vi "String To Float_csm.vi"(2 "Default (0)":dbl, 5 "String":string) -> (0 "Float":dbl format="%.2p", 1 "Unit String":string)   [LabVIEW 2017, in "API String Arguments Support.lvlib"]
uses:
  API String Arguments Support.lvlib
  <userlib>/_NEVSTOP/Communicable State Machine(CSM)/_Shared/CSM Shared.lvlib
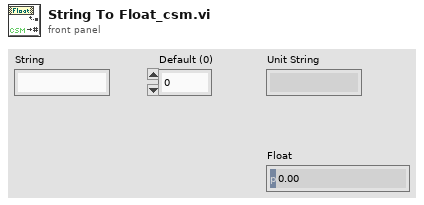
[diagram p1: front panel]
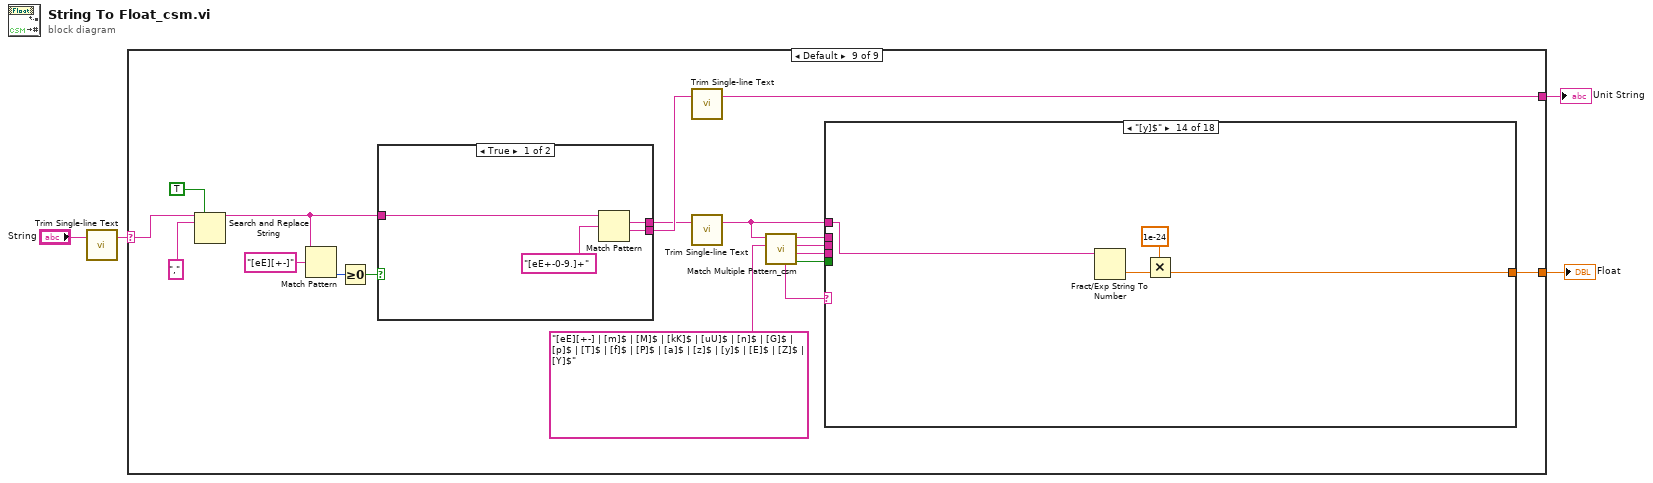
[diagram p0: block diagram]
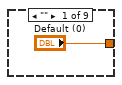
[diagram p2: hidden frame]
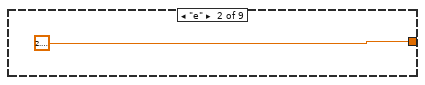
[diagram p3: hidden frame]
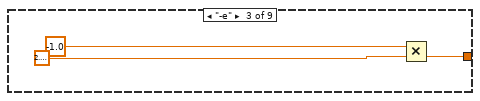
[diagram p4: hidden frame]
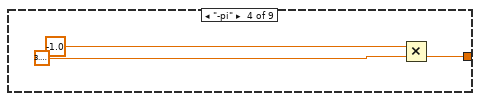
[diagram p5: hidden frame]
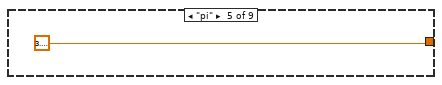
[diagram p6: hidden frame]
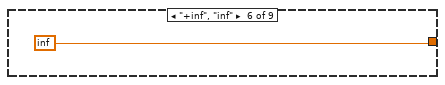
[diagram p7: hidden frame]
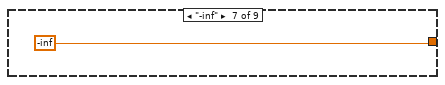
[diagram p8: hidden frame]
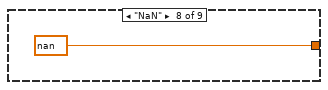
[diagram p9: hidden frame]
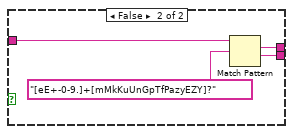
[diagram p10: hidden frame]
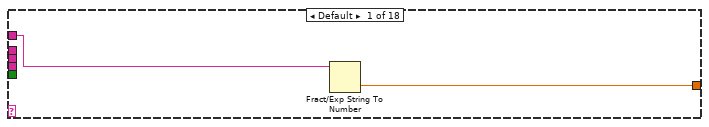
[diagram p11: hidden frame]
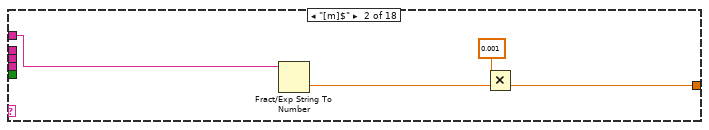
[diagram p12: hidden frame]
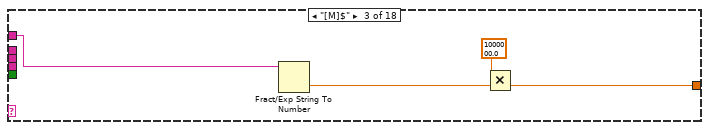
[diagram p13: hidden frame]
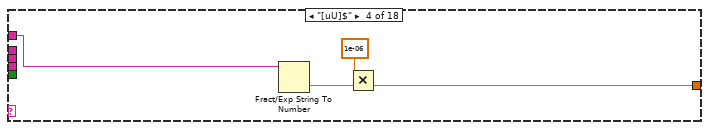
[diagram p14: hidden frame]
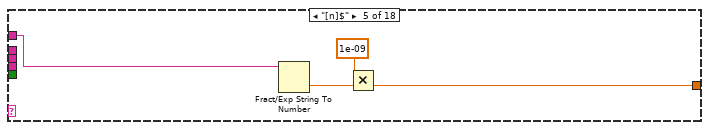
[diagram p15: hidden frame]
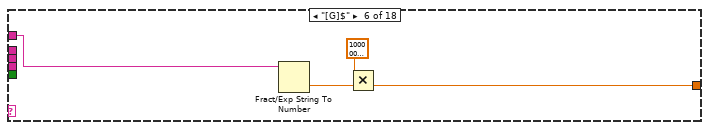
[diagram p16: hidden frame]
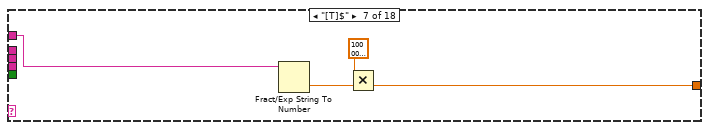
[diagram p17: hidden frame]
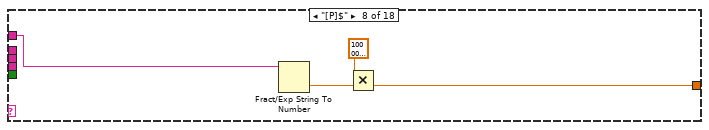
[diagram p18: hidden frame]
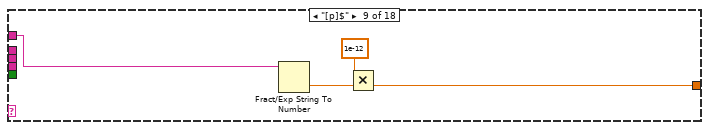
[diagram p19: hidden frame]
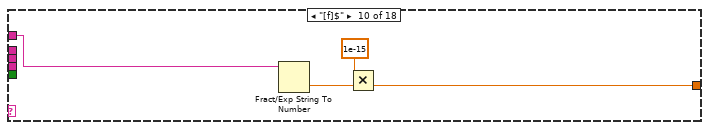
[diagram p20: hidden frame]
diagram:
  n1 = call <userlib>:"Trim Single-line Text.vi"("single-line text"="String") -> ("trimed text"=w2:string)  [unwired: 2 in]
  n2 = case shown="Default" w2 {
    selector: w2 -> [_ _ _ _ _ _ _ _ w25]
    tunnel: ["Default (0)" 2.718281828459045 w8 w11 3.141592653589793 inf -inf nan ("Default(0)") w27] -> w3
    tunnel: [_ _ _ _ _ _ _ _ w23] -> w1
    frame "" {
    }
    frame "e" {
    }
    frame "-e" {
      n3 = Multiply(x=-1.0, y=2.718281828459045) -> (x*y=w8:dbl)
    }
    frame "-pi" {
      n4 = Multiply(x=-1.0, y=3.141592653589793) -> (x*y=w11:dbl)
    }
    frame "pi" {
    }
    frame "+inf", "inf" {
    }
    frame "-inf" {
    }
    frame "NaN" {
    }
    frame Default {
      n5 = Search and Replace String(replace all?=TRUE ("replace all? (F)"), input string=w25, search string=",") -> (result string=w19:string)  [unwired: 5 in, 3 out]
      n6 = Match Pattern(string=w19, regular expression="[eE][+-]") -> (offset past match=w18:i32)  [unwired: 1 in, 3 out]
      n7 = Greater Or Equal To 0?(x=w18) -> (x >= 0?=w17:bool)
      n8 = case shown="True" w17 {
        tunnel: [w37 w41] -> w24
        tunnel: [w36 w40] -> w22
        tunnel: w19 -> [w35 w39]
        frame True {
          n9 = Match Pattern(string=w35, regular expression="[eE+-0-9.]+") -> (match substring=w36:string, after substring=w37:string)  [unwired: 1 in, 2 out]
        }
        frame False {
          n10 = Match Pattern(string=w39, regular expression="[eE+-0-9.]+[mMkKuUnGpTfPazyEZY]?") -> (match substring=w40:string, after substring=w41:string)  [unwired: 1 in, 2 out]
        }
      }
      n11 = call <userlib>:"Trim Single-line Text.vi"("single-line text"=w24) -> ("trimed text"=w23:string)  [unwired: 2 in]
      n12 = call <userlib>:"Trim Single-line Text.vi"("single-line text"=w22) -> ("trimed text"=w21:string)  [unwired: 2 in]
      n13 = call "Match Multiple Pattern_csm.vi"("regular expression"="[eE][+-] | [m]$ | [M]$ | [kK]$ | [uU]$ | [n]$ | [G]$ | [p]$ | [T]$ | [f]$ | [P]$ | [a]$ | [z]$ | [y]$ | [E]$ | [Z]$ | [Y]$", "string"=w21) -> ("Found?"=w31:bool, "after substring"=w29:string, "match substring"=w26:string, "before substring"=w28:string, "pattern matched"=w30:string)  [unwired: 5 in]
      n14 = case shown="\"[y]$\"" w30 {
        tunnel: w29 -> [_ _ _ _ _ _ _ _ _ _ _ _ _ _ _ _ _ w118]
        tunnel: w28 -> [_ _ _ _ _ _ _ _ _ _ _ _ _ _ _ _ _ w119]
        tunnel: [w43 w46 w50 w54 w58 w62 w66 w70 w74 w78 w82 w86 w90 w94 w98 w102 w106 w109] -> w27
        tunnel: w21 -> [w44 w48 w52 w56 w60 w64 w68 w72 w76 w80 w84 w88 w92 w96 w100 w104 w108 _]
        tunnel: w31 -> [_ _ _ _ _ _ _ _ _ _ _ _ _ _ _ _ _ _]
        tunnel: w26 -> [_ _ _ _ _ _ _ _ _ _ _ _ _ _ _ _ _ w117]
        frame Default {
          n15 = Fract/Exp String To Number(string=w44) -> (number=w43:dbl)  [unwired: 3 in, 1 out]
        }
        frame "[m]$" {
          n16 = Fract/Exp String To Number(string=w48) -> (number=w47:dbl)  [unwired: 3 in, 1 out]
          n17 = Multiply(x=0.001, y=w47) -> (x*y=w46:dbl)
        }
        frame "[M]$" {
          n18 = Fract/Exp String To Number(string=w52) -> (number=w51:dbl)  [unwired: 3 in, 1 out]
          n19 = Multiply(x=1000000.0, y=w51) -> (x*y=w50:dbl)
        }
        frame "[uU]$" {
          n20 = Fract/Exp String To Number(string=w56) -> (number=w55:dbl)  [unwired: 3 in, 1 out]
          n21 = Multiply(x=1e-06, y=w55) -> (x*y=w54:dbl)
        }
        frame "[n]$" {
          n22 = Fract/Exp String To Number(string=w60) -> (number=w59:dbl)  [unwired: 3 in, 1 out]
          n23 = Multiply(x=1e-09, y=w59) -> (x*y=w58:dbl)
        }
        frame "[G]$" {
          n24 = Fract/Exp String To Number(string=w64) -> (number=w63:dbl)  [unwired: 3 in, 1 out]
          n25 = Multiply(x=1000000000.0, y=w63) -> (x*y=w62:dbl)
        }
        frame "[T]$" {
          n26 = Fract/Exp String To Number(string=w68) -> (number=w67:dbl)  [unwired: 3 in, 1 out]
          n27 = Multiply(x=1000000000000.0, y=w67) -> (x*y=w66:dbl)
        }
        frame "[P]$" {
          n28 = Fract/Exp String To Number(string=w72) -> (number=w71:dbl)  [unwired: 3 in, 1 out]
          n29 = Multiply(x=1000000000000000.0, y=w71) -> (x*y=w70:dbl)
        }
        frame "[p]$" {
          n30 = Fract/Exp String To Number(string=w76) -> (number=w75:dbl)  [unwired: 3 in, 1 out]
          n31 = Multiply(x=1e-12, y=w75) -> (x*y=w74:dbl)
        }
        frame "[f]$" {
          n32 = Fract/Exp String To Number(string=w80) -> (number=w79:dbl)  [unwired: 3 in, 1 out]
          n33 = Multiply(x=1e-15, y=w79) -> (x*y=w78:dbl)
        }
        frame "[kK]$" {
          n34 = Fract/Exp String To Number(string=w84) -> (number=w83:dbl)  [unwired: 3 in, 1 out]
          n35 = Multiply(x=1000.0, y=w83) -> (x*y=w82:dbl)
        }
        frame "[a]$" {
          n36 = Fract/Exp String To Number(string=w88) -> (number=w87:dbl)  [unwired: 3 in, 1 out]
          n37 = Multiply(x=1e-18, y=w87) -> (x*y=w86:dbl)
        }
        frame "[z]$" {
          n38 = Fract/Exp String To Number(string=w92) -> (number=w91:dbl)  [unwired: 3 in, 1 out]
          n39 = Multiply(x=1e-21, y=w91) -> (x*y=w90:dbl)
        }
        frame "[y]$" {
          n40 = Fract/Exp String To Number(string=w96) -> (number=w95:dbl)  [unwired: 3 in, 1 out]
          n41 = Multiply(x=1e-24, y=w95) -> (x*y=w94:dbl)
        }
        frame "[E]$" {
          n42 = Fract/Exp String To Number(string=w100) -> (number=w99:dbl)  [unwired: 3 in, 1 out]
          n43 = Multiply(x=1e+18, y=w99) -> (x*y=w98:dbl)
        }
        frame "[Z]$" {
          n44 = Fract/Exp String To Number(string=w104) -> (number=w103:dbl)  [unwired: 3 in, 1 out]
          n45 = Multiply(x=1e+21, y=w103) -> (x*y=w102:dbl)
        }
        frame "[Y]$" {
          n46 = Fract/Exp String To Number(string=w108) -> (number=w107:dbl)  [unwired: 3 in, 1 out]
          n47 = Multiply(x=1e+24, y=w107) -> (x*y=w106:dbl)
        }
        frame "[eE][+-]" {
          (unwired) 0.0123  # DBL
          n48 = Fract/Exp String To Number(string=w119) -> (number=w111:dbl)  [unwired: 3 in, 1 out]
          n49 = Concatenate Strings(w117, w118) -> (w116:string)
          n50 = Match Pattern(string=w116, regular expression="[eE]") -> (after substring=w114:string)  [unwired: 1 in, 3 out]
          n51 = Decimal String To Number(string=w114) -> (number=w113:i32)  [unwired: 2 in, 1 out]
          n52 = To Double Precision Float(number=w113) -> (double precision float=w112:dbl)
          n53 = Power Of 10(x=w112) -> (10^x=w110:dbl)
          n54 = Multiply(x=w111, y=w110) -> (x*y=w109:dbl)
        }
      }
    }
  }
  "Float" <- w3
  "Unit String" <- w1
